vi "FL_map COA single side.vi"(0 "xlh":dbl, 1 "weight":dbl, 5 "area":dbl, 7 "coa_x":dbl, 9 "x_l":dbl, 11 "x_r":dbl, 12 "x0":dbl, 13 "x1":dbl, 14 "x2":dbl, 15 "x3":dbl) -> (6 "area":dbl, 8 "coa_x":dbl)   [LabVIEW 2020, in "NI_Fuzzy_Logic_API.lvlib"]
uses:
  <vilib>/addons/Fuzzy Logic/NI_Fuzzy_Logic_API.lvlib
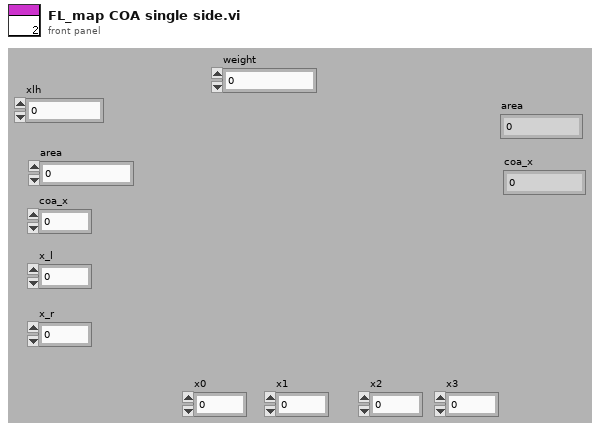
[diagram p1: front panel]
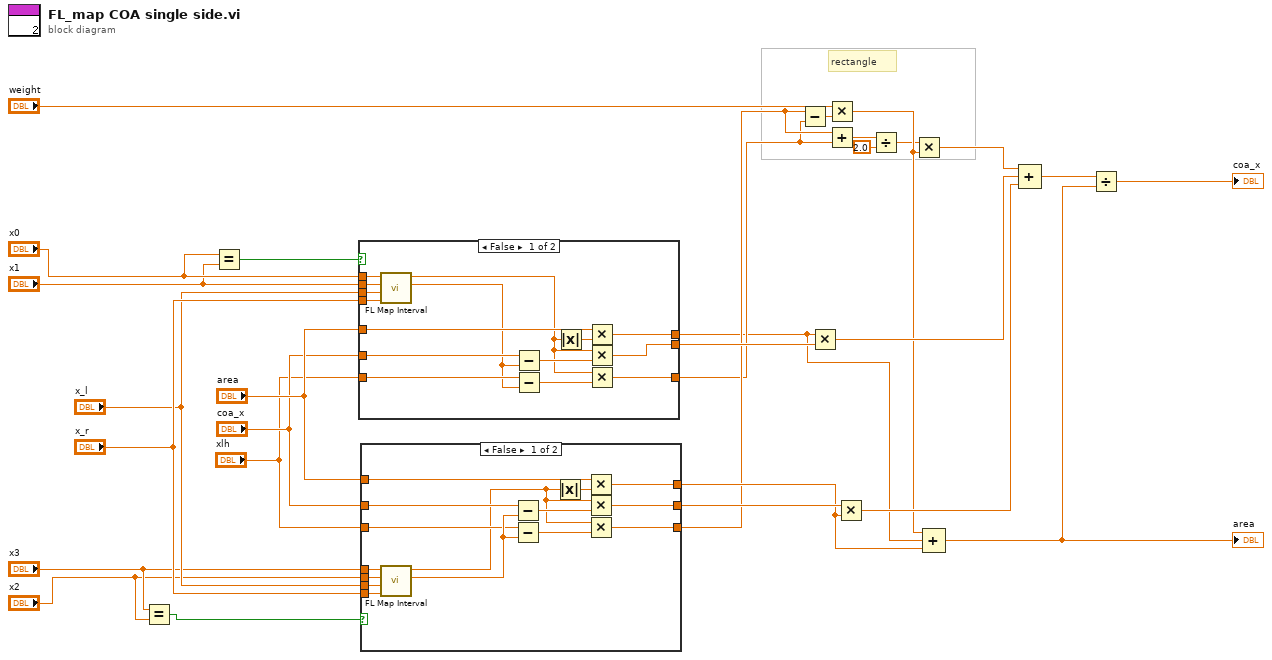
[diagram p0: block diagram]
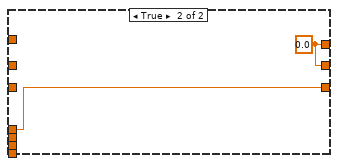
[diagram p2: hidden frame]
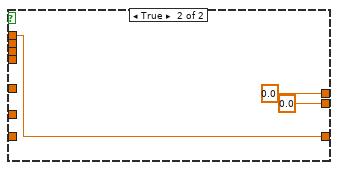
[diagram p3: hidden frame]
diagram:
  # "rectangle"
  n1 = Equal?(x="x3", y="x2") -> (x = y?=w1:bool)
  n2 = Equal?(x="x0", y="x1") -> (x = y?=w4:bool)
  n3 = case shown="False" w4 {
    tunnel: [w44 0.0] -> w25
    tunnel: "area" -> [w43 _]
    tunnel: "coa_x" -> [w42 _]
    tunnel: "x_r" -> [w39 _]
    tunnel: "x_l" -> [w38 _]
    tunnel: "x1" -> [w37 _]
    tunnel: "x0" -> [w36 w47]
    tunnel: "xlh" -> [w34 _]
    tunnel: [w31 w47] -> w8
    tunnel: [w30 0.0] -> w7
    frame False {
      n4 = call <vilib>:"FL Map Interval.vi"("x1"=w39, "x0"=w38, "b"=w37, "a"=w36) -> ("m"=w33:dbl, "k"=w32:dbl)  [unwired: 6 out]
      n5 = Subtract(x=w42, y=w33) -> (x-y=w41:dbl)
      n6 = Subtract(x=w34, y=w33) -> (x-y=w35:dbl)
      n7 = Absolute Value(x=w32) -> (abs(x)=w40:dbl)
      n8 = Multiply(x=w43, y=w40) -> (x*y=w30:dbl)
      n9 = Multiply(x=w32, y=w41) -> (x*y=w44:dbl)
      n10 = Multiply(x=w32, y=w35) -> (x*y=w31:dbl)
    }
    frame True {
    }
  }
  n11 = case shown="False" w1 {
    tunnel: "area" -> [w62 _]
    tunnel: "coa_x" -> [w61 _]
    tunnel: "x_r" -> [w60 _]
    tunnel: "x_l" -> [w59 _]
    tunnel: [w57 w63] -> w19
    tunnel: [w55 w63] -> w18
    tunnel: "x3" -> [w54 w64]
    tunnel: "x2" -> [w53 _]
    tunnel: [w50 w64] -> w10
    tunnel: "xlh" -> [w49 _]
    frame False {
      n12 = call <vilib>:"FL Map Interval.vi"("x1"=w60, "x0"=w59, "b"=w53, "a"=w54) -> ("m"=w51:dbl, "k"=w48:dbl)  [unwired: 6 out]
      n13 = Subtract(x=w61, y=w51) -> (x-y=w56:dbl)
      n14 = Subtract(x=w49, y=w51) -> (x-y=w52:dbl)
      n15 = Absolute Value(x=w48) -> (abs(x)=w58:dbl)
      n16 = Multiply(x=w62, y=w58) -> (x*y=w55:dbl)
      n17 = Multiply(x=w48, y=w56) -> (x*y=w57:dbl)
      n18 = Multiply(x=w48, y=w52) -> (x*y=w50:dbl)
    }
    frame True {
      w63 = 0.0
    }
  }
  n19 = Subtract(x=w10, y=w8) -> (x-y=w12:dbl)
  n20 = Multiply(x=w7, y=w25) -> (x*y=w27:dbl)
  n21 = Multiply(x="weight", y=w12) -> (x*y=w17:dbl)
  n22 = Add(x=w10, y=w8) -> (x+y=w13:dbl)
  n23 = Multiply(x=w19, y=w18) -> (x*y=w26:dbl)
  n24 = Divide(x=w13, y=2.0) -> (x/y=w15:dbl)
  n25 = Multiply(x=w15, y=w17) -> (x*y=w16:dbl)
  n26 = Compound Arithmetic op=ADD(w17, w7, w18) -> (w28:dbl)
  "area" <- w28
  n27 = Compound Arithmetic op=ADD(w16, w27, w26) -> (w24:dbl)
  n28 = Divide(x=w24, y=w28) -> (x/y=→"coa_x":dbl)
